vi "MapJoystick.vi"() -> (2 "Joystick Map":T1[](array[typedef]), 3 "Joysticks":T2[](array[typedef]))   [LabVIEW 2015]
uses:
  <vilib>/Rock Robotics/WPI/Joystick/WPI_JoystickDevRef.ctl
  <vilib>/Rock Robotics/WPI/Joystick/WPI_JoystickDeviceEnum.ctl
  JoystickMap.ctl
  JoystickMappingNamesTypeDef.ctl
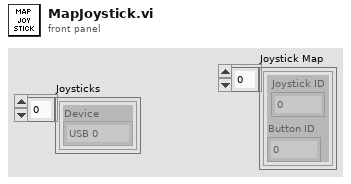
[diagram p1: front panel]
types:
  T1 = typedef "JoystickMap.ctl" = cluster{"Button ID":dbl, "Joystick ID":dbl}
  T2 = typedef "WPI_JoystickDevRef.ctl" = cluster{"Device":T3}
  T3 = typedef "WPI_JoystickDeviceEnum.ctl" = enum16{"USB 0", "USB 1", "USB 2", "USB 3", "USB 4", "USB 5"}
  T4 = typedef "JoystickMappingNamesTypeDef.ctl" = enum16{"Shoot Button", "Retrieve Button", "Arm Control", "High Gear", "Low Gear", "Enable PTO", "Disable PTO", "PortC Control", "PortC Up", "PortC Down", "Lift Control", "Drive VBus", "Override Arm Limits", "TWP Control", "TWP Final Pos"}
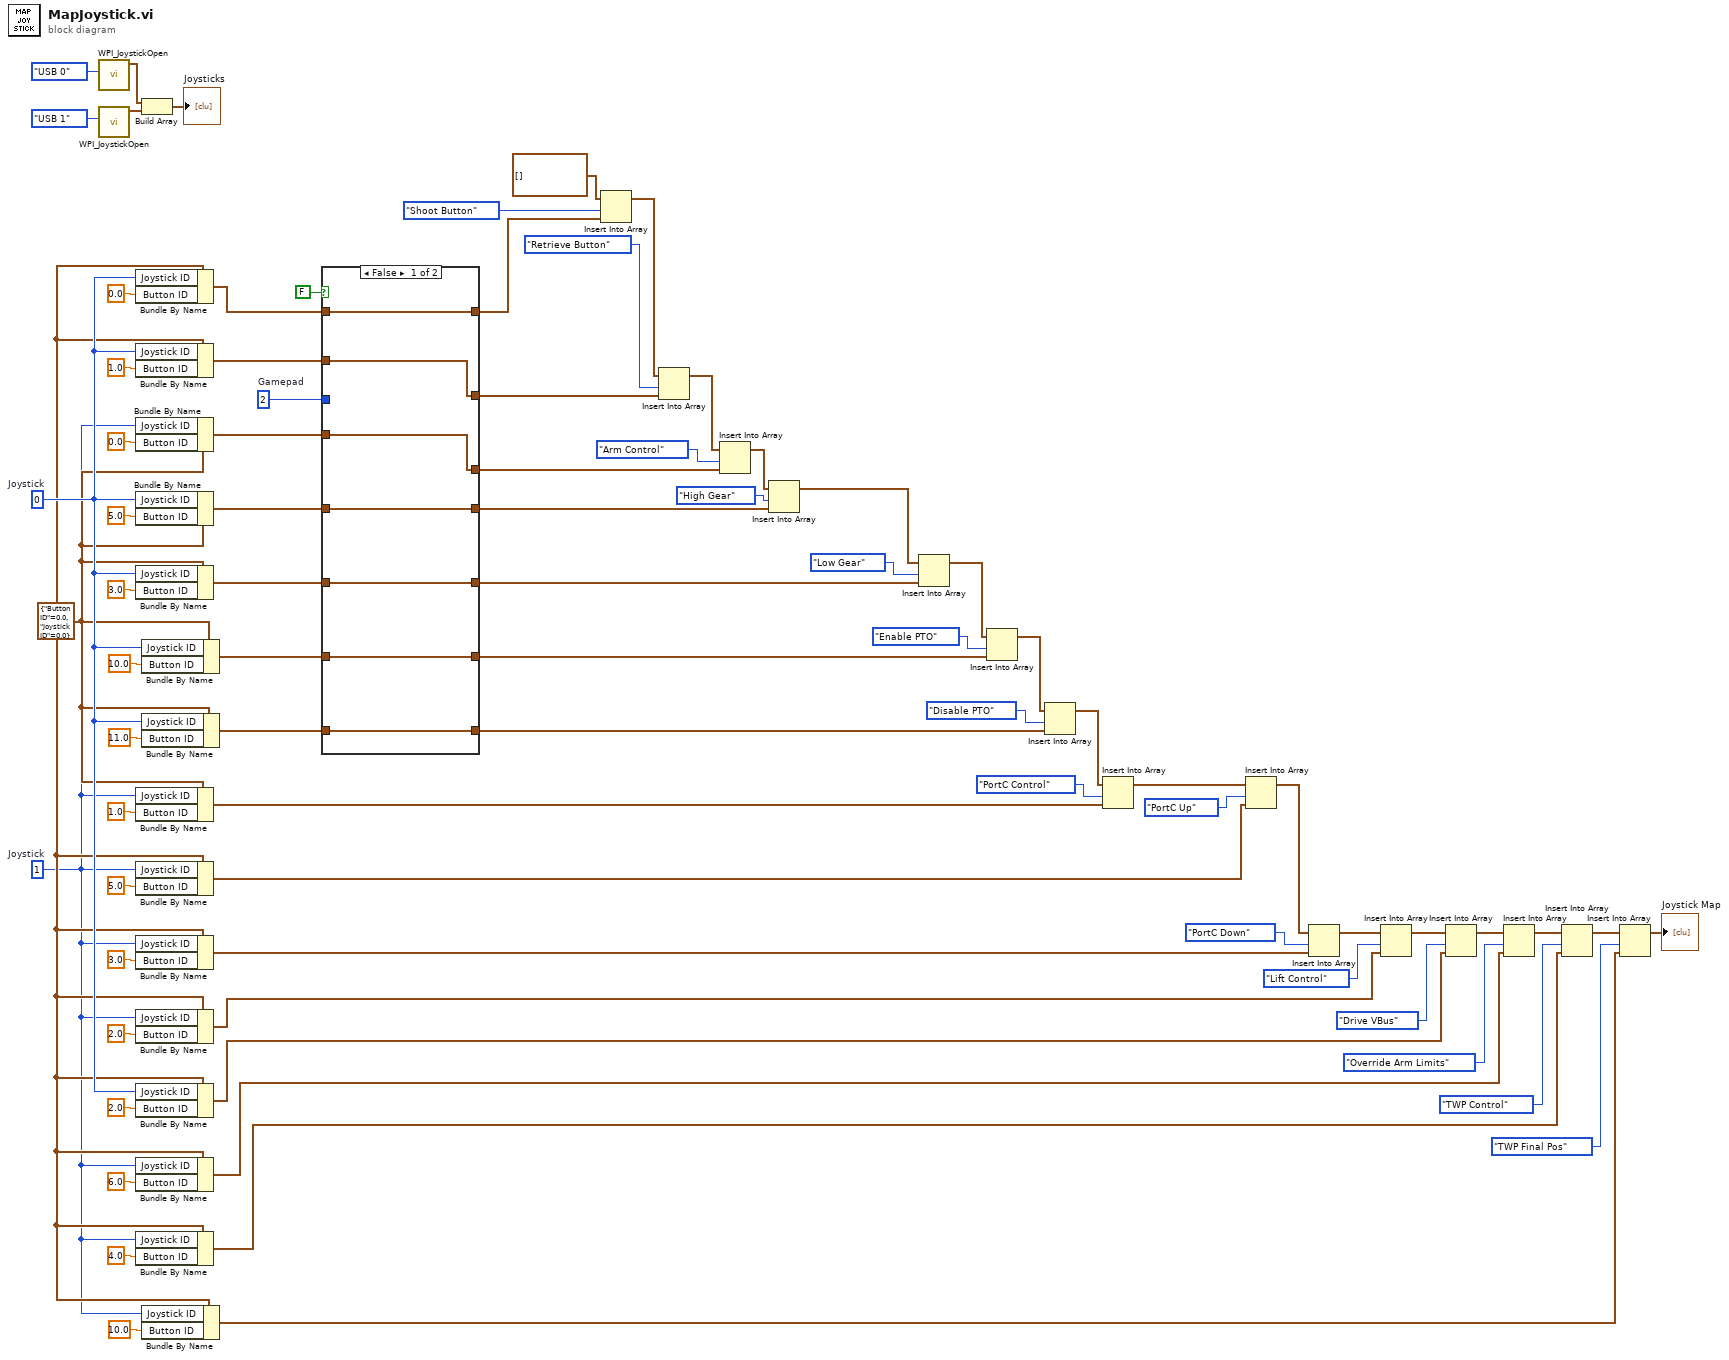
[diagram p0: block diagram]
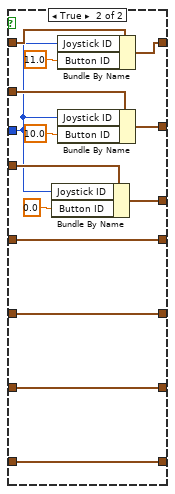
[diagram p2: hidden frame]
diagram:
  w5 = 1  # Joystick
  w44 = 2  # Gamepad
  w6 = T1 {"Button ID"=0.0, "Joystick ID"=0.0} ("Joystick Map")
  w22 = 0  # Joystick
  n1 = call <vilib>:"WPI_JoystickOpen.vi"("JoystickDevice"=WPI_JoystickDeviceEnum."USB 0") -> ("JoystickDevRef"=w58:T2)  [unwired: 10 in]
  n2 = call <vilib>:"WPI_JoystickOpen.vi"("JoystickDevice"=WPI_JoystickDeviceEnum."USB 1") -> ("JoystickDevRef"=w38:T2)  [unwired: 10 in]
  n3 = Bundle By Name(cluster=w6, "Joystick ID"=w22, "Button ID"=0.0) -> (w56:T1)
  n4 = Bundle By Name(cluster=w6, "Joystick ID"=w22, "Button ID"=1.0) -> (w53:T1)
  n5 = Bundle By Name(cluster=w6, "Joystick ID"=w5, "Button ID"=0.0) -> (w52:T1)
  n6 = Bundle By Name(cluster=w6, "Joystick ID"=w22, "Button ID"=5.0) -> (w50:T1)
  n7 = Bundle By Name(cluster=w6, "Joystick ID"=w22, "Button ID"=3.0) -> (w47:T1)
  n8 = Bundle By Name(cluster=w6, "Joystick ID"=w5, "Button ID"=1.0) -> (w39:T1)
  n9 = Bundle By Name(cluster=w6, "Joystick ID"=w5, "Button ID"=5.0) -> (w28:T1)
  n10 = Bundle By Name(cluster=w6, "Joystick ID"=w5, "Button ID"=3.0) -> (w27:T1)
  n11 = Bundle By Name(cluster=w6, "Joystick ID"=w5, "Button ID"=2.0) -> (w23:T1)
  n12 = Bundle By Name(cluster=w6, "Joystick ID"=w22, "Button ID"=2.0) -> (w19:T1)
  n13 = Bundle By Name(cluster=w6, "Joystick ID"=w5, "Button ID"=6.0) -> (w12:T1)
  n14 = Bundle By Name(cluster=w6, "Joystick ID"=w5, "Button ID"=4.0) -> (w9:T1)
  n15 = Build Array(w58, w38) -> (→"Joysticks":T2[])
  n16 = Bundle By Name(cluster=w6, "Joystick ID"=w22, "Button ID"=10.0) -> (w16:T1)
  n17 = Bundle By Name(cluster=w6, "Joystick ID"=w22, "Button ID"=11.0) -> (w17:T1)
  n18 = Bundle By Name(cluster=w6, "Joystick ID"=w5, "Button ID"=10.0) -> (w3:T1)
  n19 = case shown="False" FALSE {
    tunnel: w56 -> [w85 w97]
    tunnel: [w85 w98] -> w55
    tunnel: [w84 w96] -> w54
    tunnel: w53 -> [w84 w95]
    tunnel: w52 -> [w83 w93]
    tunnel: [w83 w89] -> w51
    tunnel: w50 -> [w82 w91]
    tunnel: [w82 w91] -> w49
    tunnel: [w81 w90] -> w48
    tunnel: w47 -> [w81 w90]
    tunnel: [w80 w87] -> w46
    tunnel: w16 -> [w80 w87]
    tunnel: w17 -> [w79 w86]
    tunnel: [w79 w86] -> w45
    tunnel: w44 -> [_ w92]
    frame False {
    }
    frame True {
      n20 = Bundle By Name(cluster=w93, "Joystick ID"=w92, "Button ID"=0.0) -> (w89:T1)
      n21 = Bundle By Name(cluster=w97, "Joystick ID"=w92, "Button ID"=11.0) -> (w98:T1)
      n22 = Bundle By Name(cluster=w95, "Joystick ID"=w92, "Button ID"=10.0) -> (w96:T1)
    }
  }
  n23 = Insert Into Array(array=T1[] [], index=JoystickMappingNamesTypeDef."Shoot Button" ("Joystick Button Names"), new element=w55) -> (w75:T1[])
  n24 = Insert Into Array(array=w75, index=JoystickMappingNamesTypeDef."Retrieve Button" ("Joystick Button Names"), new element=w54) -> (w72:T1[])
  n25 = Insert Into Array(array=w72, index=JoystickMappingNamesTypeDef."Arm Control" ("Joystick Button Names"), new element=w51) -> (w35:T1[])
  n26 = Insert Into Array(array=w35, index=JoystickMappingNamesTypeDef."High Gear" ("Joystick Button Names"), new element=w49) -> (w67:T1[])
  n27 = Insert Into Array(array=w67, index=JoystickMappingNamesTypeDef."Low Gear" ("Joystick Button Names"), new element=w48) -> (w61:T1[])
  n28 = Insert Into Array(array=w61, index=JoystickMappingNamesTypeDef."Enable PTO" ("Joystick Button Names"), new element=w46) -> (w62:T1[])
  n29 = Insert Into Array(array=w62, index=JoystickMappingNamesTypeDef."Disable PTO" ("Joystick Button Names"), new element=w45) -> (w40:T1[])
  n30 = Insert Into Array(array=w40, index=JoystickMappingNamesTypeDef."PortC Control" ("Joystick Button Names"), new element=w39) -> (w33:T1[])
  n31 = Insert Into Array(array=w33, index=JoystickMappingNamesTypeDef."PortC Up" ("Joystick Button Names"), new element=w28) -> (w34:T1[])
  n32 = Insert Into Array(array=w34, index=JoystickMappingNamesTypeDef."PortC Down" ("Joystick Button Names"), new element=w27) -> (w25:T1[])
  n33 = Insert Into Array(array=w25, index=JoystickMappingNamesTypeDef."Lift Control" ("Joystick Button Names"), new element=w23) -> (w21:T1[])
  n34 = Insert Into Array(array=w21, index=JoystickMappingNamesTypeDef."Drive VBus" ("Joystick Button Names"), new element=w19) -> (w15:T1[])
  n35 = Insert Into Array(array=w15, index=JoystickMappingNamesTypeDef."Override Arm Limits" ("Joystick Button Names"), new element=w12) -> (w8:T1[])
  n36 = Insert Into Array(array=w8, index=JoystickMappingNamesTypeDef."TWP Control" ("Joystick Button Names"), new element=w9) -> (w2:T1[])
  n37 = Insert Into Array(array=w2, index=JoystickMappingNamesTypeDef."TWP Final Pos" ("Joystick Button Names"), new element=w3) -> (→"Joystick Map":T1[])
